vi "imageClicked.vi"(8 "error in (no error)":errorcluster, 10 "Point":T1, 11 "ImageStreamViewer in":refnum<class "ImageStreamViewer.lvclass">) -> (0 "error out":errorcluster, 3 "ImageStreamViewer out":refnum<class "ImageStreamViewer.lvclass">)   [LabVIEW 2011, in "Views.lvlib" / "Camera.lvlib" / "ImageStreamViewer.lvclass"]
uses:
  ImageStreamViewer.lvclass
  <vilib>/Utility/miscctls.llb/LVPoint32TypeDef.ctl
  ImageStreamViewer.lvclass/ImageStreamViewer.ctl
panel:
  # "the user has clicked the image.\nAt the coorindate of Point.\nWe need to decide what kind of \ninteraction the user requires. \n\nDrawing a ROI,changing tool, or \nrepositioning the cross."
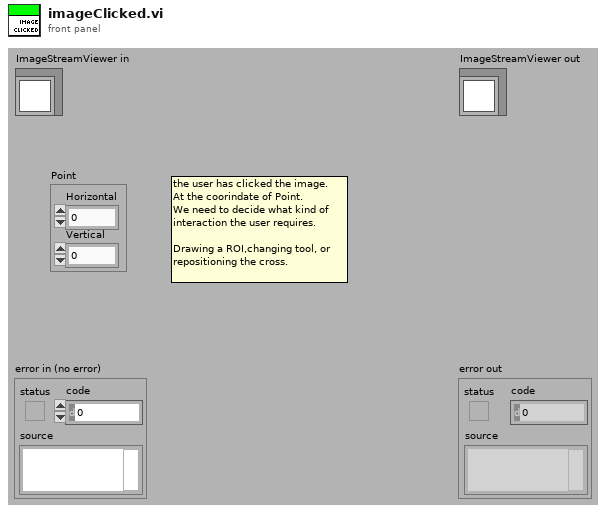
[diagram p1: front panel]
types:
  T1 = typedef "LVPoint32TypeDef.ctl" = cluster{"Horizontal":i32, "Vertical":i32}
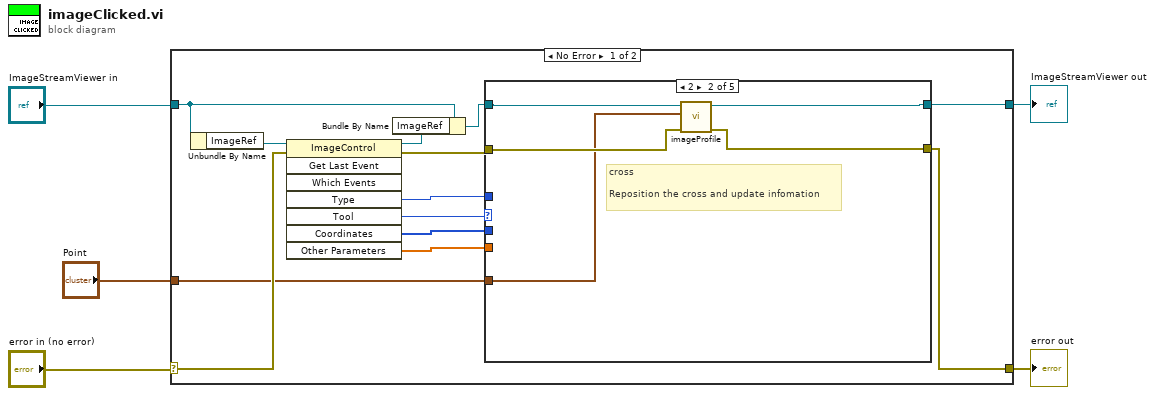
[diagram p0: block diagram]
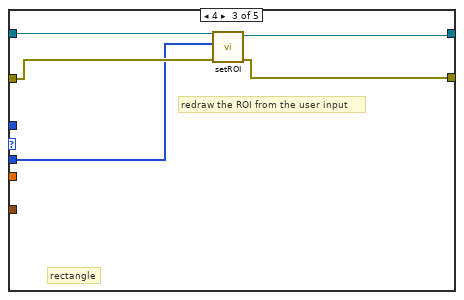
[diagram p3: hidden frame]
diagram:
  n1 = case shown="No Error" "error in (no error)" {
    selector: "error in (no error)" -> [w17 w36]
    tunnel: [w10 w36] -> w4
    tunnel: [w16 w35] -> w2
    tunnel: "ImageStreamViewer in" -> [w8 w35]
    tunnel: "Point" -> [w6 _]
    frame No Error {
      n2 = Unbundle By Name(w8) -> ("ImageRef"=w18:refnum<vi>)
      n3 = invoke on="Invoke Node" class="ImageControl" method="Get Last Event"(reference=w18, error in=w17) -> (reference out=w9:refnum<vi>, error out=w14:errorcluster, "Type"=w13:i32, "Tool"=w15:i32, "Coordinates"=w12:i32[], "Other Parameters"=w11:sgl[])  [unwired: 6 in, 2 out]
      n4 = Bundle By Name(cluster=w8, "ImageRef"=w9) -> (w7:refnum<class "ImageStreamViewer.lvclass">)
      n5 = case shown="2" w15 {
        tunnel: [w20 w24 w29 w32 w34] -> w16
        tunnel: w7 -> [w20 w25 w30 w32 w34]
        tunnel: w14 -> [w19 w23 w27 w31 w33]
        tunnel: w13 -> [_ _ _ _ _]
        tunnel: w12 -> [_ _ w26 _ _]
        tunnel: w11 -> [_ _ _ _ _]
        tunnel: [w19 w22 w28 w31 w33] -> w10
        tunnel: w6 -> [_ w21 _ _ _]
        frame 0, Default {
          # "the user selected a different tool"
          # "selection tool"
        }
        frame 2 {
          # "cross\n\nReposition the cross and update infomation"
          n6 = call "imageProfile.vi"("error in (no error)"=w23, "Point"=w21, "ImageStreamViewer in"=w25) -> ("error out"=w22:errorcluster, "ImageStreamViewer out"=w24:refnum<class "ImageStreamViewer.lvclass">)  [unwired: 7 in]
        }
        frame 4 {
          # "redraw the ROI from the user input"
          # "rectangle"
          n7 = call "setROI.vi"("error in (no error)"=w27, "Coordinates"=w26, "ImageStreamViewer in"=w30) -> ("error out"=w28:errorcluster, "ImageStreamViewer out"=w29:refnum<class "ImageStreamViewer.lvclass">)  [unwired: 7 in]
        }
        frame 10 {
          # "the user selected a different tool\nthe zoom tool"
          # "zoom"
        }
        frame 11 {
          # "The user selected the pan tool"
          # "pan"
        }
      }
    }
    frame Error {
    }
  }
  "error out" <- w4
  "ImageStreamViewer out" <- w2
